vi "Position to Direction.vi"(8 "Starting Coords":T1, 10 "Position":T1, 11 "Goal":T1) -> (0 "Direction":T2, 3 "Distance":i32)   [LabVIEW 2017, in "Dauntless.lvclass"]
uses:
  Dauntless.lvclass
  Type Defs/Direction Enum.ctl
  Coords Cluster.ctl
  SubVIs/Read-Only Globals.vi
  SubVIs/Globals (private).vi
  Square/Square.lvclass
  Type Defs/SB Type Defs.lvlib
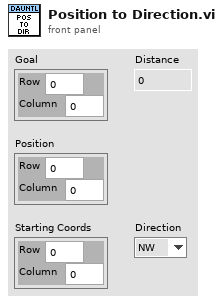
[diagram p1: front panel]
types:
  T1 = typedef "Dauntless.lvclass/Coords Cluster.ctl" = cluster{"Row":i32, "Column":i32}
  T2 = typedef "SB Type Defs.lvlib/Direction Enum.ctl" = enum16{"NW", "N", "NE", "E", "SE", "S", "SW", "W"}
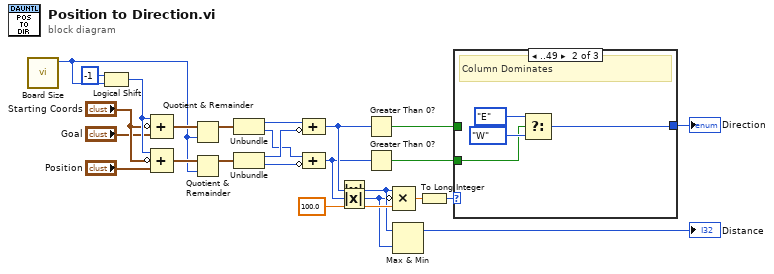
[diagram p0: block diagram]
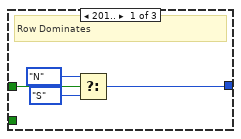
[diagram p2: hidden frame]
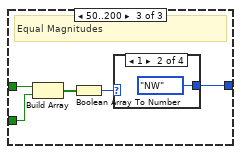
[diagram p3: hidden frame]
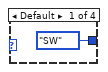
[diagram p4: hidden frame]
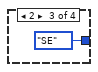
[diagram p5: hidden frame]
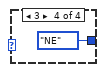
[diagram p6: hidden frame]
diagram:
  n1 = call "Board Size.vi"() -> ("Board Size"=w1:i32)  [unwired: 11 in]
  n2 = Logical Shift(y=i16 -1, x=w1) -> (x << y=w21:i32)
  n3 = Compound Arithmetic op=ADD(w21, invert "Starting Coords", "Goal") -> (w22:T1)
  n4 = Compound Arithmetic op=ADD(w21, invert "Starting Coords", "Position") -> (w23:T1)
  n5 = Quotient & Remainder(x=w22, y=w1) -> (x-y*floor(x/y)=w18:T1)  [unwired: 1 out]
  n6 = Quotient & Remainder(x=w23, y=w1) -> (x-y*floor(x/y)=w17:T1)  [unwired: 1 out]
  n7 = Unbundle(w18) -> ("Row"=w16:i32, "Column"=w13:i32)
  n8 = Unbundle(w17) -> ("Row"=w15:i32, "Column"=w14:i32)
  n9 = Compound Arithmetic op=ADD(w16, invert w15) -> (w9:i32)
  n10 = Compound Arithmetic op=ADD(w13, invert w14) -> (w8:i32)
  n11 = Absolute Value(x=w9) -> (abs(x)=w4:i32)
  n12 = Absolute Value(x=w8) -> (abs(x)=w3:i32)
  n13 = Greater Than 0?(x=w9) -> (x > 0?=w7:bool)
  n14 = Greater Than 0?(x=w8) -> (x > 0?=w6:bool)
  n15 = Compound Arithmetic op=MULTIPLY(w4, invert w3, 100.0 ("value")) -> (w11:dbl)
  n16 = Max & Min(x=w4, y=w3) -> (max(x,y)=→"Distance":i32)  [unwired: 1 out]
  n17 = To Long Integer(number=w11) -> (32bit integer=w10:i32)
  n18 = case shown="..49" w10 {
    tunnel: w7 -> [w29 _ w38]
    tunnel: w6 -> [_ w30 w37]
    tunnel: [w26 w31 w34] -> w5
    frame 201.. {
      # "Row Dominates"
      n19 = Select(t=Direction_Enum."N" ("Direction"), s=w29, f=Direction_Enum."S" ("Direction")) -> (s? t:f=w26:T2)
    }
    frame ..49 {
      # "Column Dominates"
      n20 = Select(t=Direction_Enum."E" ("Direction"), s=w30, f=Direction_Enum."W" ("Direction")) -> (s? t:f=w31:T2)
    }
    frame 50..200 {
      # "Equal Magnitudes"
      n21 = Build Array(w38, w37) -> (w36:bool[])
      n22 = Boolean Array To Number(Boolean array=w36) -> (number=w35:u32)
      n23 = case shown="1" w35 {
        tunnel: [Direction_Enum."SW" ("Direction") Direction_Enum."NW" ("Direction") Direction_Enum."SE" ("Direction") Direction_Enum."NE" ("Direction")] -> w34
        frame Default {
        }
        frame 1 {
        }
        frame 2 {
        }
        frame 3 {
        }
      }
    }
  }
  "Direction" <- w5
